vi "Get Process IDs.vi"(11 "Process in":refnum<class "Process.lvclass">) -> (2 "Process IDs":string[](array[string]), 3 "Process out":refnum<class "Process.lvclass">)   [LabVIEW 2019, in "TimingDRV Engine.lvlib" / "Process.lvclass"]
uses:
  Process.lvclass
  Process.lvclass/Process.ctl
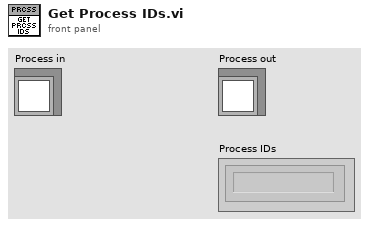
[diagram p1: front panel]
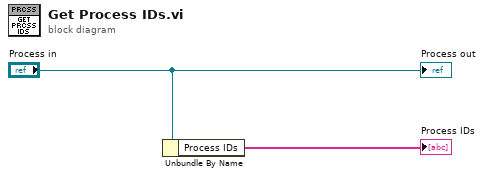
[diagram p0: block diagram]
diagram:
  n1 = Unbundle By Name("Process in") -> ("Process IDs"=→"Process IDs":string[])
  "Process out" <- "Process in"
